vi "Scale And Set Data Array.vi"(8 "Error In":errorcluster, 10 "Data Array":dbl[](array[numeric]), 11 "Graph In":refnum<class "Graph.lvclass">) -> (0 "Error Out":errorcluster, 3 "Graph Out":refnum<class "Graph.lvclass">)   [LabVIEW 2019, in "Graph.lvclass"]
uses:
  Graph.lvclass
  <vilib>/ErrorRing/Error Ring.xnode
  <vilib>/Utility/error.llb/Error Cluster From Error Code.vi
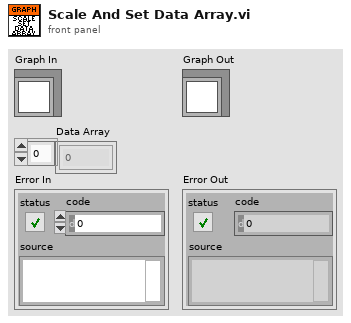
[diagram p1: front panel]
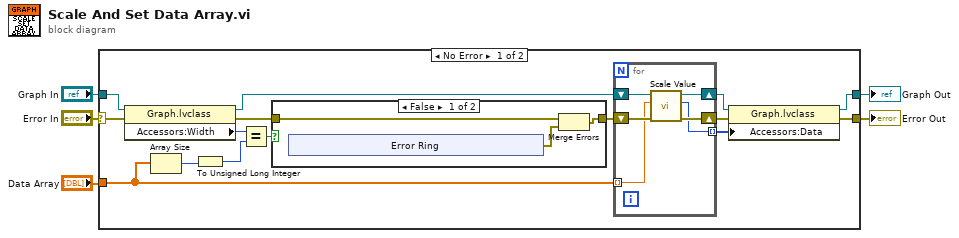
[diagram p0: block diagram]
diagram:
  n1 = case shown="No Error" "Error In" {
    selector: "Error In" -> [w15 w37]
    tunnel: "Graph In" -> [w14 w36]
    tunnel: [w19 w37] -> w3
    tunnel: [w20 w36] -> w2
    tunnel: "Data Array" -> [w13 _]
    frame No Error {
      n2 = property class="Graph.lvclass"(reference=w14, error in=w15) -> (reference out=w11:refnum<class "Graph.lvclass">, error out=w10:errorcluster, "Accessors:Width"=w12:u32)
      n3 = Array Size(array=w13) -> (size(s)=w9:i32)
      n4 = To Unsigned Long Integer(number=w9) -> (unsigned 32bit integer=w8:u32)
      n5 = Equal?(x=w12, y=w8) -> (x = y?=w6:bool)
      n6 = case shown="False" w6 {
        tunnel: w10 -> [w23 w29]
        tunnel: [w22 w29] -> w7
        frame False {
          n7 = xnode "Error Ring"() -> ("error out"=w21:errorcluster)
          n8 = Merge Errors(w23, w21) -> (w22:errorcluster)
        }
        frame True {
        }
      }
      n9 = for {
        tunnel: w13 -> [w33] mode=indexing
        shift-right: [w32] -> w18
        shift-left: w7 -> [w35]
        shift-right: [w31] -> w17
        shift-left: w11 -> [w34]
        tunnel: [w30] -> w16 mode=indexing
        n10 = call "Scale Value.vi"("Error In"=w35, "Value"=w33, "Graph In"=w34) -> ("Error Out"=w32:errorcluster, "Scaled Value"=w30:i32, "Graph Out"=w31:refnum<class "Graph.lvclass">)  [unwired: 6 in]
      }
      n11 = property class="Graph.lvclass"(reference=w17, error in=w18, "Accessors:Data"=w16) -> (reference out=w20:refnum<class "Graph.lvclass">, error out=w19:errorcluster)
    }
    frame Error {
    }
  }
  "Graph Out" <- w2
  "Error Out" <- w3
